vi "N4_X01.vi"(4 "error in":T15, 7 "Command":T16) -> (0 "error out":T15, 3 "Response":T13)   [LabVIEW 2018]
uses:
  MOKO_LabViewLibrary/MokoLowLevel/MokoLowLovelControl/MLLC_Command.ctl
  MOKO_LabViewLibrary/MokoLowLevel/MokoLowLovelControl/MLLC_Error.ctl
  MOKO_LabViewLibrary/MokoLowLevel/MokoLowLovelControl/MLLC_Mode.ctl
  MOKO_LabViewLibrary/MokoLowLevel/MokoLowLovelControl/MLLC_Response.ctl
  MOKO_LabViewLibrary/MokoLowLevel/MokoLowLovelControl/MLLC_DriverName.ctl
  MOKO_LabViewLibrary/MokoLowLevel/MokoLowLovelControl/MLLC_Request.ctl
  MOKO_LabViewLibrary/MokoLowLevel/MokoLowLovelControl/MLLC_ErrorCode.ctl
  MOKO_LabViewLibrary/MokoLowLevel/MokoLowLovelControl/MLLC_ResponseInit.ctl
  MOKO_LabViewLibrary/MokoLowLevel/MokoLowLovelControl/MLLC_ConnectCluster.ctl
  MOKO_LabViewLibrary/MokoLowLevel/MokoLowLovelControl/MLLC_InterfaceType.ctl
  MOKO_LabViewLibrary/MokoLowLevel/MokoLowLovelControl/MLLC_OpenedSession.ctl
  MOKO_LabViewLibrary/MokoLowLevel/MokoLowLovelControl/MLLC_InterfaceSettings.ctl
  MOKO_LabViewLibrary/MokoLowLevel/MokoLowLovelControl/MLLC_InterfaceKind.ctl
  MOKO_LabViewLibrary/MokoLowLevel/MokoLowLovelControl/MLLC_Boolean.ctl
  MOKO_LabViewLibrary/MokoLowLevel/MokoLowLovelControl/MLLC_Delay.ctl
panel:
  in  "Settings":T8={"Saved Data"=variant, "Permanent data"={"Connect"={"InterfaceType"=enum."VISA", "OpenedSession"="COM1", "InterfaceSettings"={"Interface"=enum."RS232", "EOS 4 read"=enum."LF (\\n)", "EOS 4 write"=enum."LF (\\n)", "TMO, ms"=10000, "Sett"=variant(cluster{"Baud Rate":u32, "Data Bits":u16, "Parity":u16, "Stop Bits":u16, "Flow Control":u16, "Eho":bool} {"Baud Rate"=75, "Data Bits"=0, "Parity"=0, "Stop Bits"=0, "Flow Control"=0, "Eho"=FALSE})}}, "RangeAuto"=TRUE, "SwitchOFF"=TRUE, "Range"=0.0}}
  in  "ResponseInit":T9="N4-101"
  in  "Error Code":T10=5470
  in  "Request":T11="IDN?"
  in  "Driver Name":T12="N4_101"
  in  "Mode":T14=enum."Check"
  # "Í4-X01"
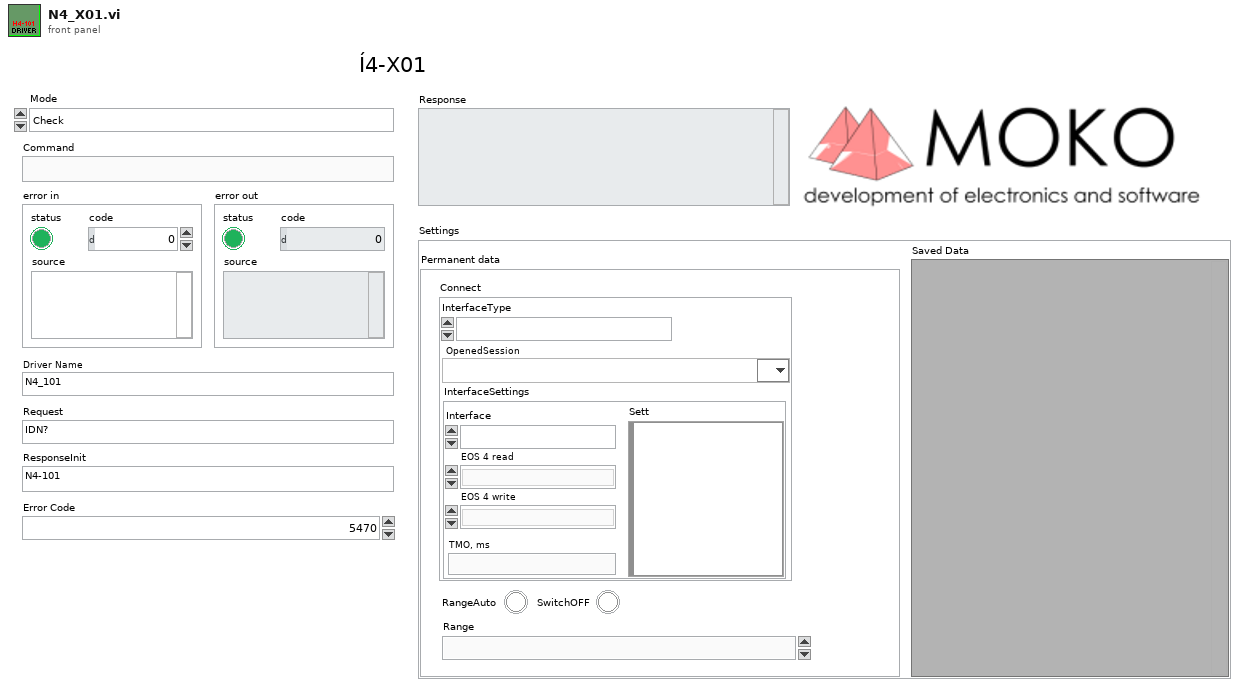
[diagram p1: front panel]
types:
  T1 = typedef "MLLC_ConnectCluster.ctl" = cluster{"InterfaceType":T2, "OpenedSession":T3, "InterfaceSettings":T4}
  T2 = typedef "MLLC_InterfaceType.ctl" = enum16{"VISA", "Prologix USB-GPIB"}
  T3 = typedef "MLLC_OpenedSession.ctl" = refnum<visa-resource-name>
  T4 = typedef "MLLC_InterfaceSettings.ctl" = cluster{"Interface":T5, "EOS 4 read":enum16{"Default (=EOS 4 write)", "CR (\\r)", "LF (\\n)", "None"}, "EOS 4 write":enum16{"CR+LF (\\r\\n)", "CR (\\r)", "LF (\\n)", "None"}, "TMO, ms":i32, "Sett":variant}
  T5 = typedef "MLLC_InterfaceKind.ctl" = enum16{"RS232", "GPIB", "USB", "Ethernet", "another"}
  T6 = typedef "MLLC_Boolean.ctl" = bool
  T7 = typedef "MLLC_Delay.ctl" = dbl
  T8 = cluster{"Saved Data":variant, "Permanent data":cluster{"Connect":T1, "RangeAuto":T6, "SwitchOFF":T6, "Range":T7}}
  T9 = typedef "MLLC_ResponseInit.ctl" = string
  T10 = typedef "MLLC_ErrorCode.ctl" = u32
  T11 = typedef "MLLC_Request.ctl" = string
  T12 = typedef "MLLC_DriverName.ctl" = string
  T13 = typedef "MLLC_Response.ctl" = string
  T14 = typedef "MLLC_Mode.ctl" = enum16{"get", "set", "close", "Init", "Check"}
  T15 = typedef "MLLC_Error.ctl" = errorcluster
  T16 = typedef "MLLC_Command.ctl" = string
  T17 = cluster{"Connect":T1, "RangeAuto":T6, "SwitchOFF":T6, "Range":T7}
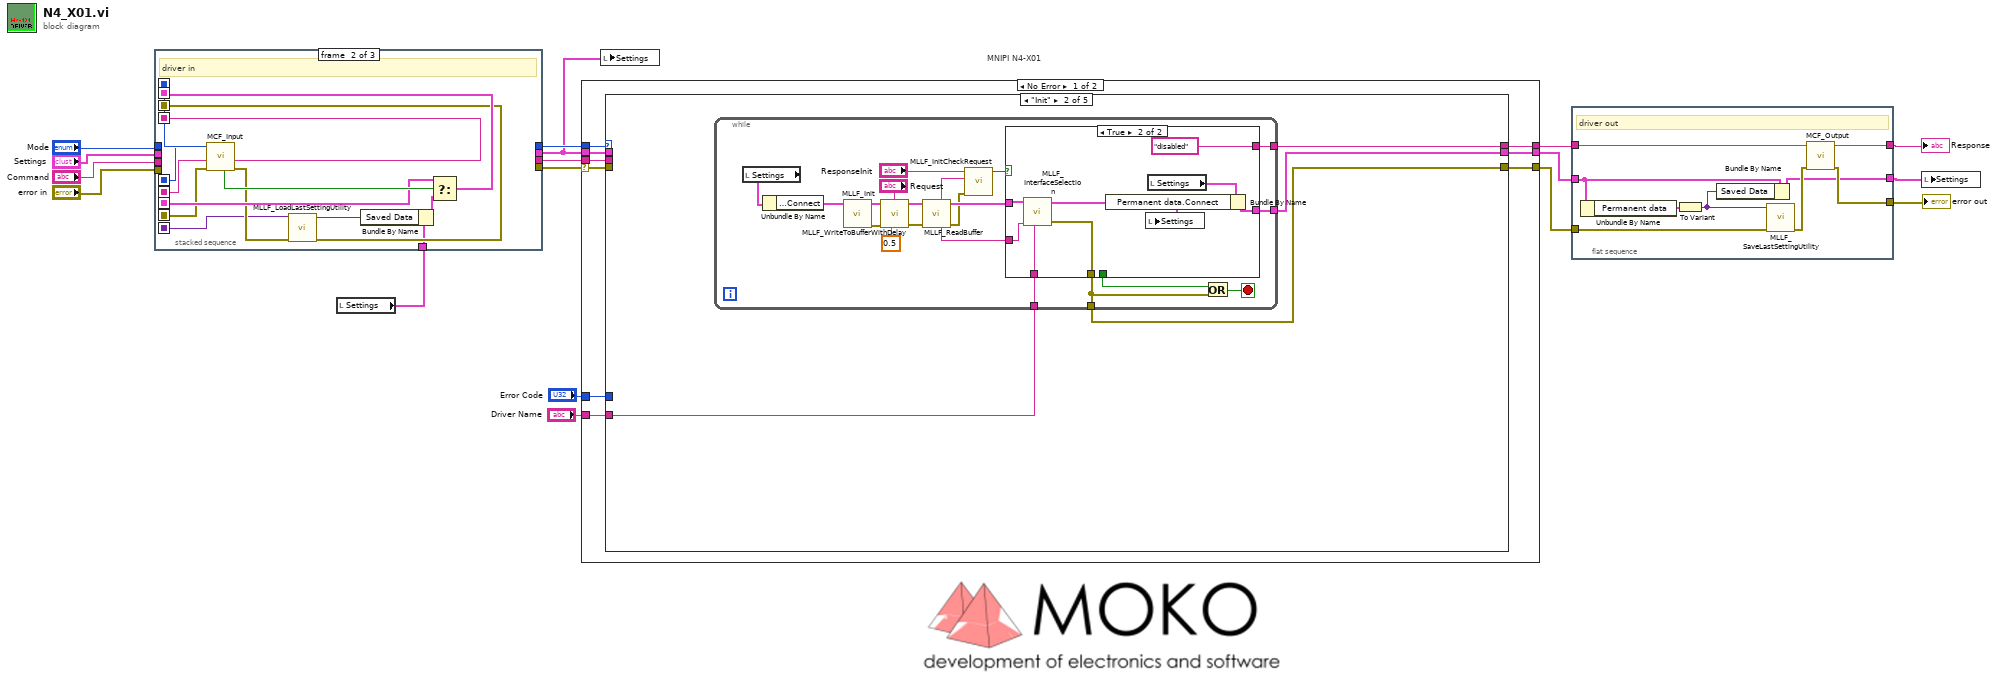
[diagram p0: block diagram]
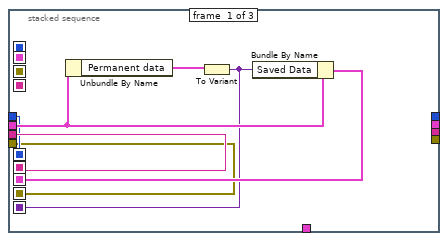
[diagram p2: hidden frame]
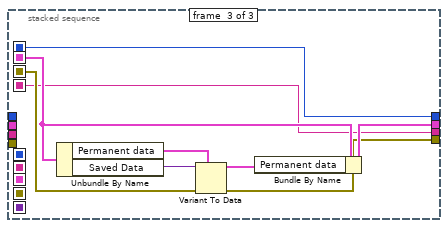
[diagram p3: hidden frame]
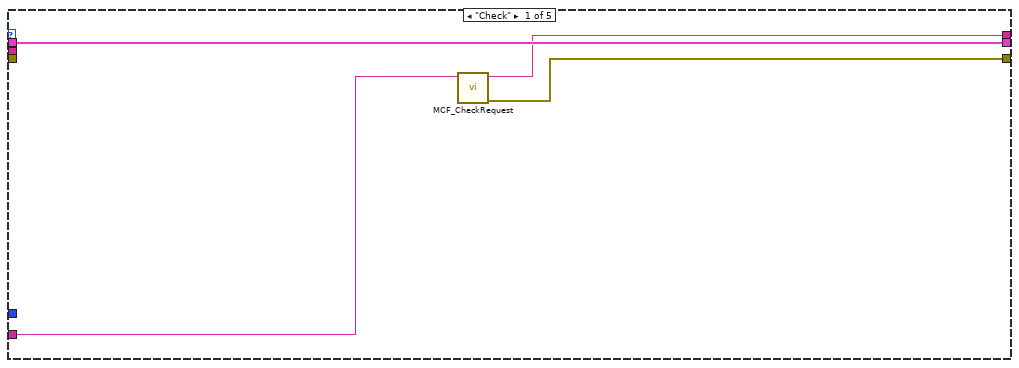
[diagram p4: hidden frame]
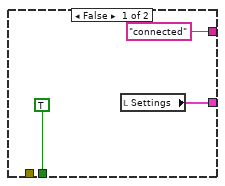
[diagram p5: hidden frame]
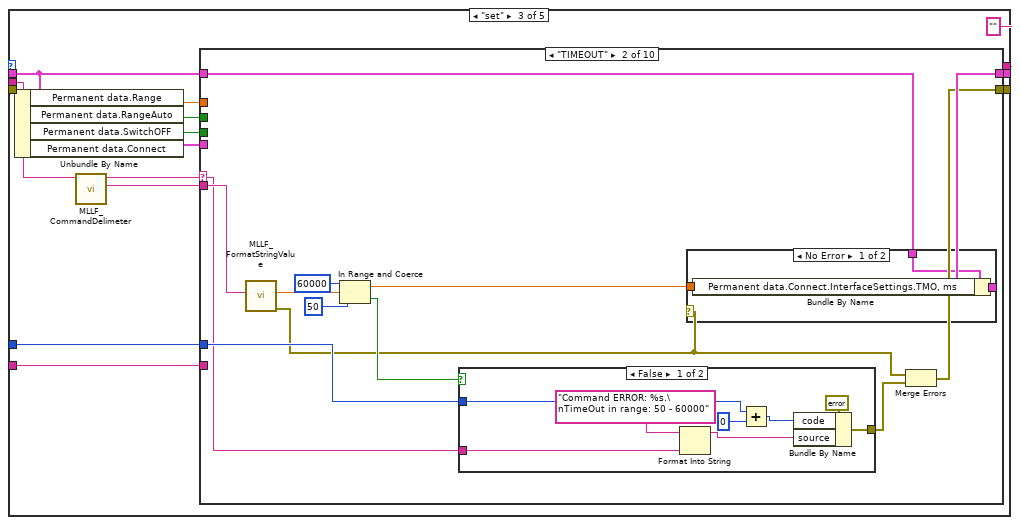
[diagram p6: hidden frame]
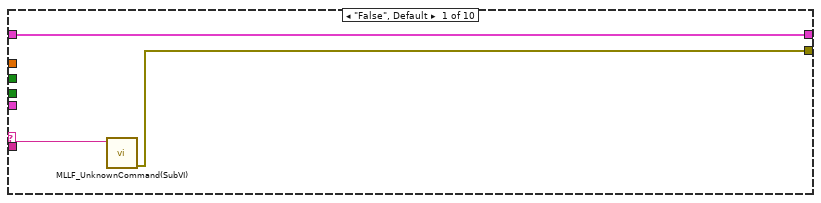
[diagram p7: hidden frame]
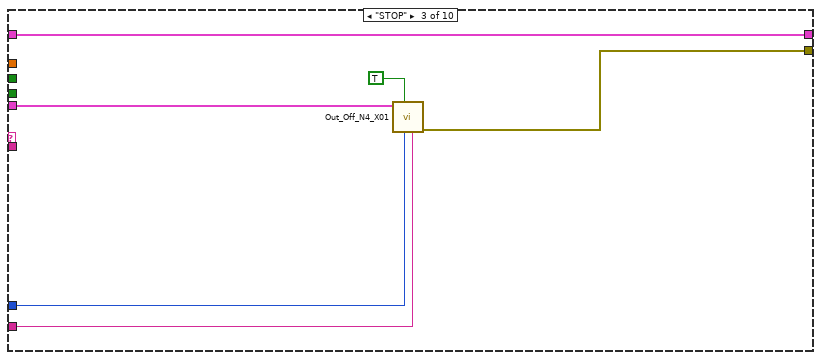
[diagram p10: hidden frame]
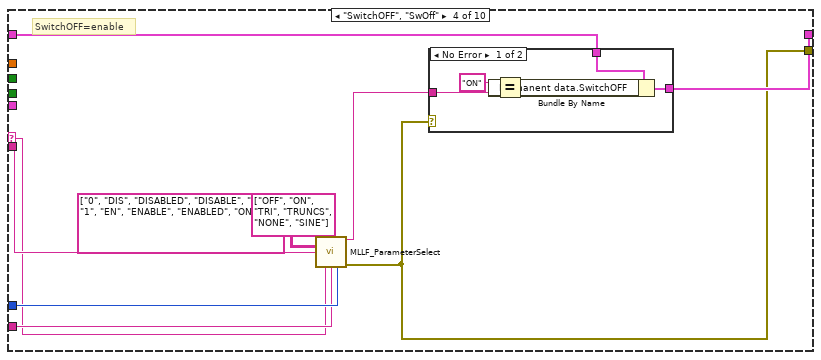
[diagram p11: hidden frame]
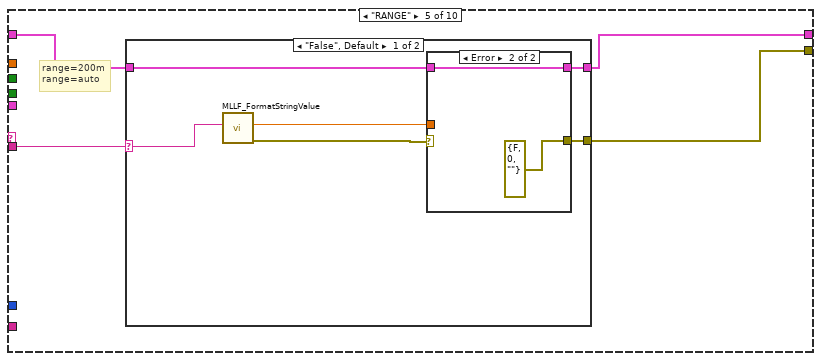
[diagram p13: hidden frame]
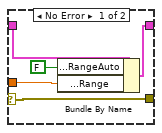
[diagram p14: hidden frame]
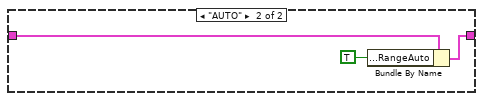
[diagram p15: hidden frame]
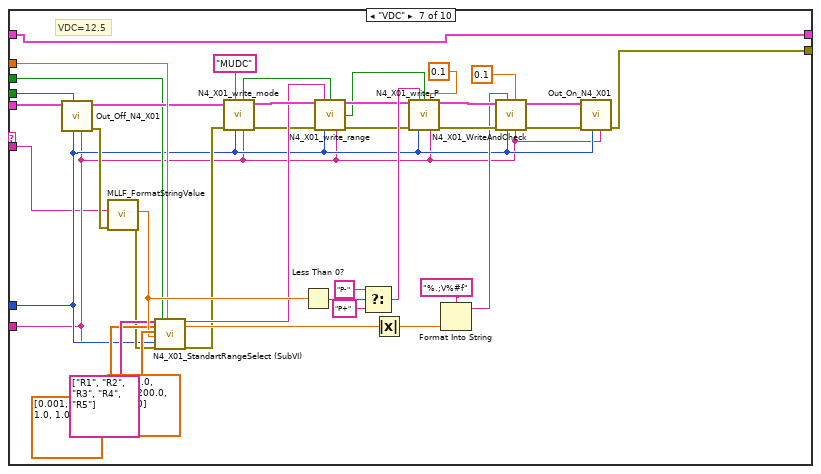
[diagram p17: hidden frame]
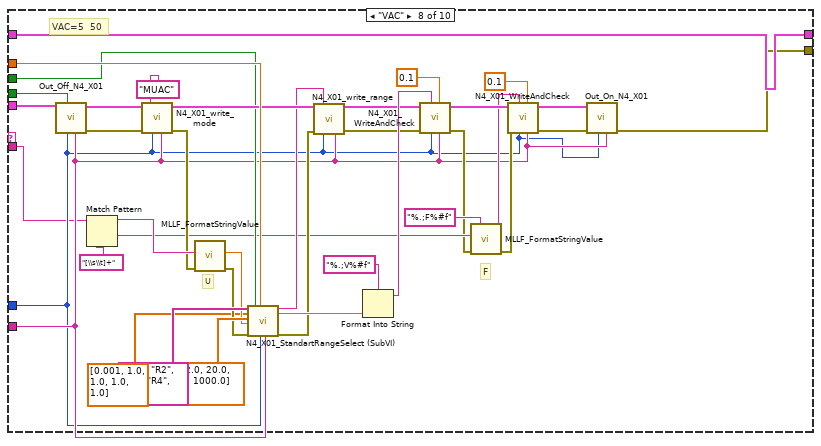
[diagram p18: hidden frame]
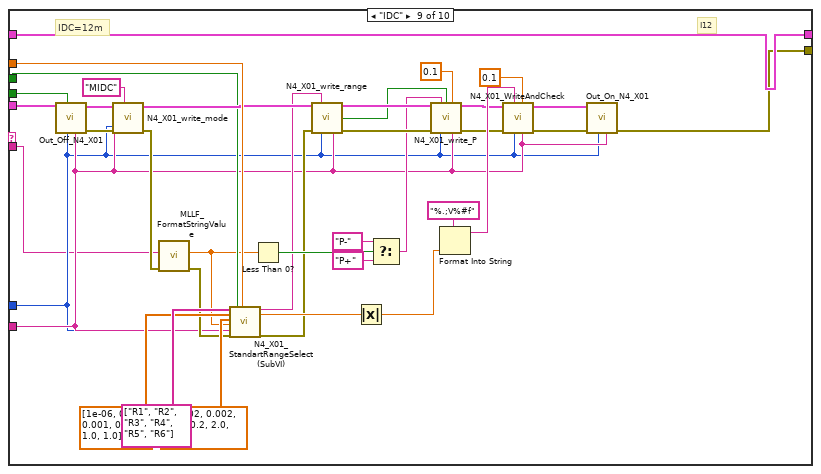
[diagram p19: hidden frame]
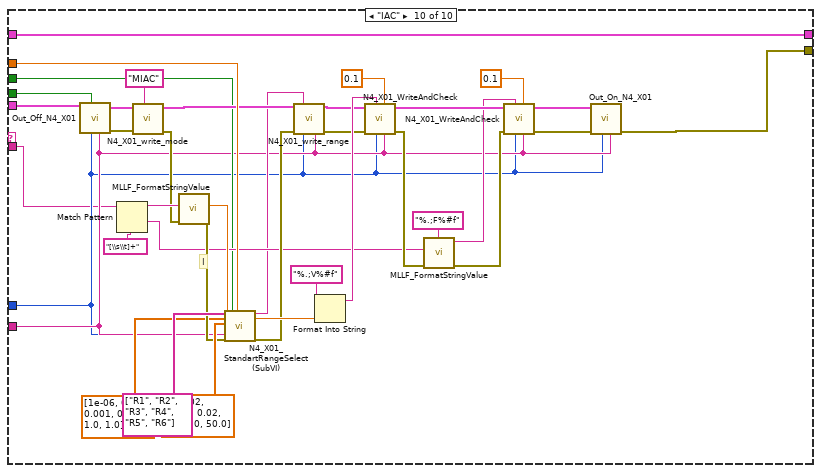
[diagram p20: hidden frame]
diagram:
  # "MNIPI N4-X01"
  n1 = local read "Settings"() -> (w7:T8)
  n2 = stacked-sequence {
    seq-local: [w20 _ _] -> [_ w36 _]
    seq-local: [w19 _ _] -> [_ w37 _]
    seq-local: [w22 _ _] -> [_ w32 _]
    seq-local: [w18 _ _] -> [_ w31 _]
    seq-local: [w21 _ _] -> [_ w27 _]
    seq-local: [_ w28 _] -> [_ _ w44]
    seq-local: [_ w38 _] -> [_ _ w41]
    seq-local: [_ w35 _] -> [_ _ w40]
    seq-local: [_ w34 _] -> [_ _ w45]
    tunnel: "Command" -> [w20 _ _]
    tunnel: "Mode" -> [w19 _ _]
    tunnel: "error in" -> [w18 _ _]
    tunnel: "Settings" -> [w23 _ _]
    tunnel: w7 -> [_ w26 _]
    tunnel: [_ _ w40] -> w9
    tunnel: [_ _ w43] -> w10
    tunnel: [_ _ w42] -> w8
    tunnel: [_ _ w41] -> w11
    frame #0 {
      n3 = Unbundle By Name(w23) -> ("Permanent data"=w24:T17)
      n4 = To Variant(anything=w24) -> (Variant=w21:variant)
      n5 = Bundle By Name(cluster=w23, "Saved Data"=w21) -> (w22:T8)
    }
    frame #1 {
      # "driver in"
      n6 = call "MCF_Input.vi"("Error In"=w31, "Command in"=w36, "Mode in"=w37) -> ("Error Out"=w30:errorcluster, "Command out"=w35:string, "Mode out"=w38:T14, "Boolean"=w33:bool)  [unwired: 5 in]
      n7 = call "MLLF_LoadLastSettingUtility.vi"("Error In"=w30, "Save data in"=w27) -> ("Error Out"=w28:errorcluster, "Save data out"=w25:variant)  [unwired: 8 in]
      n8 = Bundle By Name(cluster=w26, "Saved Data"=w25) -> (w29:T8)
      n9 = Select(t=w32, s=w33, f=w29) -> (s? t:f=w34:T8)
    }
    frame #2 {
      n10 = Unbundle By Name(w45) -> ("Permanent data"=w46:T17, "Saved Data"=w39:variant)
      n11 = Variant To Data(error in=w44, type=w46, Variant=w39) -> (data=w47:T17, error out=w42:errorcluster)
      n12 = Bundle By Name(cluster=w45, "Permanent data"=w47) -> (w43:T8)
    }
  }
  n13 = case shown="No Error" w8 {
    selector: w8 -> [w52 w371]
    tunnel: [w54 w371] -> w4
    tunnel: w11 -> [w56 _]
    tunnel: [w55 "" ("String")] -> w6
    tunnel: w9 -> [w53 _]
    tunnel: w10 -> [w49 w370]
    tunnel: "Error Code" -> [w51 _]
    tunnel: "Driver Name" -> [w50 _]
    tunnel: [w48 w370] -> w5
    frame No Error {
      n14 = case shown="\"Init\"" w56 {
        tunnel: [w58 w64 "" ("String") w333 "" ("String")] -> w55
        tunnel: [w59 w62 w97 w332 w367] -> w54
        tunnel: w53 -> [_ _ w107 w343 _]
        tunnel: w52 -> [_ _ _ _ _]
        tunnel: w51 -> [_ _ w106 w340 _]
        tunnel: w50 -> [w57 w61 w103 w339 _]
        tunnel: w49 -> [w60 _ w105 w342 w366]
        tunnel: [w60 w63 w104 w341 w366] -> w48
        frame "Check" {
          n15 = call "MCF_CheckRequest.vi"("Driver Name"=w57) -> ("Error Out"=w59:errorcluster, "Output String"=w58:string)  [unwired: 9 in]
        }
        frame "Init" {
          n16 = while {
            tunnel: [w76] -> w62
            tunnel: [w68] -> w63
            tunnel: [w67] -> w64
            tunnel: w61 -> [w66]
            stop <- w74 stop-if-true
            n17 = local read "Settings"() -> (w83:T8)
            n18 = Unbundle By Name(w83) -> ("Permanent data.Connect"=w77:T1)
            n19 = call "MLLF_Init.vi"("DriverConnect in"=w77) -> ("Error Out"=w79:errorcluster, "DriverConnect out"=w78:T1)  [unwired: 7 in]
            n20 = call "MLLF_WriteToBufferWithDelay.vi"("Delay Time ( 0,05 s)"=0.5 ("Delay Time (s)"), "Command"="Request", "Error In"=w79, "DriverConnect in"=w78) -> ("Error Out"=w72:errorcluster, "DriverConnect out"=w81:T1)  [unwired: 6 in]
            n21 = call "MLLF_ReadBuffer.vi"("Error In"=w72, "DriverConnect in"=w81) -> ("Error Out"=w70:errorcluster, "DriverConnect out"=w80:T1, "String"=w65:string)  [unwired: 6 in]
            n22 = call "MLLF_InitCheckRequest.vi"("error in (no error)"=w70, "Answer"=w65, "Response Init"="ResponseInit") -> ("Design"=w69:bool)  [unwired: 5 in, 3 out]
            n23 = case shown="True" w69 {
              tunnel: w80 -> [_ w93]
              tunnel: [_ w94] -> w76
              tunnel: [TRUE _] -> w75
              tunnel: [w84 w90] -> w68
              tunnel: ["connected" "disabled"] -> w67
              tunnel: w66 -> [_ w88]
              tunnel: w65 -> [_ w87]
              frame False {
                n24 = local read "Settings"() -> (w84:T8)
              }
              frame True {
                n25 = call "MLLF_InterfaceSelection.vi"("Driver Name"=w88, "Answer:"=w87, "DriverConnect in"=w93) -> ("error out"=w94:T15, "DriverConnect out"=w92:T1)  [unwired: 4 in, 3 out]
                n26 = local read "Settings"() -> (w91:T8)
                n27 = Bundle By Name(cluster=w91, "Permanent data.Connect"=w92) -> (w90:T8)
                n28 = local write "Settings"(w90) -> ()
              }
            }
            n29 = Or(x=w75, y=w76) -> (x .or. y?=w74:bool)
          }
        }
        frame "set" {
          n30 = Unbundle By Name(w105) -> ("Permanent data.Range"=w98:T7, "Permanent data.RangeAuto"=w99:T6, "Permanent data.SwitchOFF"=w100:T6, "Permanent data.Connect"=w101:T1)
          n31 = call "MLLF_CommandDelimeter.vi"("command with param"=w107) -> ("param 1"=w95:string, "command"=w96:string)  [unwired: 6 in, 3 out]
          n32 = case shown="\"TIMEOUT\"" w96 {
            selector: w96 -> [w109 w111 _ w142 _ _ _ _ _ _]
            tunnel: w95 -> [_ w114 _ w143 w161 _ w179 w219 w256 w295]
            tunnel: [w108 w117 w140 w146 w160 _ w180 w218 w257 w294] -> w97
            tunnel: w106 -> [_ w118 w138 w145 _ _ w183 w220 w259 w296]
            tunnel: w105 -> [w110 w122 w141 w148 w159 w178 w217 w254 w292 w330]
            tunnel: [w110 w123 w141 w147 w158 w178 w217 w254 w292 w330] -> w104
            tunnel: w101 -> [_ _ w137 _ _ _ w201 w255 w293 w331]
            tunnel: w103 -> [_ _ w139 w144 _ _ w182 w221 w260 w297]
            tunnel: w100 -> [_ _ _ _ _ _ w200 w246 w287 w321]
            tunnel: w99 -> [_ _ _ _ _ _ w194 w232 w267 w302]
            tunnel: w98 -> [_ _ _ _ _ _ w202 w238 w279 w313]
            frame "False", Default {
              n33 = call "MLLF_UnknownCommand(SubVI).vi"("Unknown command"=w109) -> ("error out"=w108:errorcluster)  [unwired: 10 in]
            }
            frame "TIMEOUT" {
              n34 = call "MLLF_FormatStringValue.vi"("String Value"=w114) -> ("error out"=w112:T15, "number"=w113:dbl)  [unwired: 8 in, 1 out]
              n35 = In Range and Coerce(upper limit=60000, x=w113, lower limit=50) -> (coerced(x)=w119:dbl, In Range?=w115:bool)
              n36 = case shown="False" w115 {
                tunnel: [w130 _] -> w116
                tunnel: w118 -> [w129 _]
                tunnel: w111 -> [w128 _]
                frame False {
                  n37 = Format Into String(format string="Command ERROR: %s.\nTimeOut in range: 50 - 60000", w128) -> (resulting string=w132:string)  [unwired: 2 in, 1 out]
                  n38 = Add(x=w129, y=0) -> (x+y=w133:T10)
                  n39 = Bundle By Name(cluster=errorcluster {"status"=TRUE, "code"=0, "source"=""} ("error out"), "code"=w133, "source"=w132) -> (w130:errorcluster)
                }
                frame True {
                }
              }
              n40 = case shown="No Error" w112 {
                tunnel: [w126 w127] -> w123
                tunnel: w122 -> [w125 w127]
                tunnel: w119 -> [w124 _]
                frame No Error {
                  n41 = Bundle By Name(cluster=w125, "Permanent data.Connect.InterfaceSettings.TMO, ms"=w124) -> (w126:T8)
                }
                frame Error {
                }
              }
              n42 = Merge Errors(w112, w116) -> (w117:errorcluster)
            }
            frame "STOP" {
              n43 = call "Out_Off_N4_X01.vi"("Driver Name"=w139, "Error Code"=w138, "SwitchOFF"=TRUE, "DriverConnect in"=w137) -> ("error out"=w140:T15)  [unwired: 6 in, 1 out]
            }
            frame "SwitchOFF", "SwOff" {
              # "SwitchOFF=enable"
              n44 = call "MLLF_ParameterSelect.vi"("Command to equipment"=string[] ["OFF", "ON", "TRI", "TRUNCS", "NONE", "SINE"] ("Parameters"), "Names"=string[][] [["0", "DIS", "DISABLED", "DISABLE", "OFF"], ["1", "EN", "ENABLE", "ENABLED", "ON"]], "Input"=w143, "Command"=w142, "Driver Name"=w144, "Error Code"=w145) -> ("Choice"=w151:string, "Error Out"=w146:errorcluster)  [unwired: 8 in]
              n45 = case shown="No Error" w146 {
                tunnel: w151 -> [w156 _]
                tunnel: w148 -> [w154 w157]
                tunnel: [w153 w157] -> w147
                frame No Error {
                  n46 = Equal?(x="ON", y=w156) -> (x = y?=w152:bool)
                  n47 = Bundle By Name(cluster=w154, "Permanent data.SwitchOFF"=w152) -> (w153:T8)
                }
                frame Error {
                }
              }
            }
            frame "RANGE" {
              # "range=200m\nrange=auto"
              n48 = case shown="\"False\", Default" w161 {
                selector: w161 -> [w167 _]
                tunnel: [w162 _] -> w160
                tunnel: [w165 w177] -> w158
                tunnel: w159 -> [w166 w176]
                frame "False", Default {
                  n49 = call "MLLF_FormatStringValue.vi"("String Value"=w167) -> ("error out"=w163:T15, "number"=w164:dbl)  [unwired: 8 in, 1 out]
                  n50 = case shown="Error" w163 {
                    selector: w163 -> [w168 _]
                    tunnel: w166 -> [w171 w174]
                    tunnel: [w170 w174] -> w165
                    tunnel: w164 -> [w169 _]
                    tunnel: [w168 errorcluster {"status"=FALSE, "code"=0, "source"=""} ("error IO")] -> w162
                    frame No Error {
                      n51 = Bundle By Name(cluster=w171, "Permanent data.RangeAuto"=FALSE ("RangeAuto"), "Permanent data.Range"=w169) -> (w170:T8)
                    }
                    frame Error {
                    }
                  }
                }
                frame "AUTO" {
                  n52 = Bundle By Name(cluster=w176, "Permanent data.RangeAuto"=TRUE ("RangeAuto")) -> (w177:T8)
                }
              }
            }
            frame "<----MAIN FUNCTIONS---->" {
            }
            frame "VDC" {
              # "VDC=12.5"
              n53 = call "Out_Off_N4_X01.vi"("Driver Name"=w182, "Error Code"=w183, "SwitchOFF"=w200, "DriverConnect in"=w201) -> ("error out"=w190:T15, "DriverConnect out"=w196:T1)  [unwired: 6 in]
              n54 = call "MLLF_FormatStringValue.vi"("error in"=w190, "String Value"=w179) -> ("error out"=w192:T15, "number"=w215:dbl)  [unwired: 7 in, 1 out]
              n55 = call "N4_X01_StandartRangeSelect (SubVI).vi"("Range Command"=string[] ["R1", "R2", "R3", "R4", "R5"] ("RangeCommand"), "Scale Array"=dbl[] [0.001, 1.0, 1.0, 1.0, 1.0] ("ScaleArray"), "Range Digit"=dbl[] [0.2, 2.0, 20.0, 200.0, 1000.0] ("RangeDigit"), "Control Point"=w215, "Error In"=w192, "RangeAuto"=w194, "Range"=w202, "Error Code"=w183, "Driver Name"=w182) -> ("Range Out"=w195:string, "Scaled value"=w213:dbl, "Error Out"=w189:errorcluster)  [unwired: 8 in]
              n56 = call "N4_X01_write_mode.vi"("Driver Name"=w182, "Error Code"=w183, "Command"="MUDC" ("String"), "error in"=w189, "DriverConnect in"=w196) -> ("error out"=w188:T15, "DriverConnect out"=w199:T1, "ModeWasChacged"=w187:T6)  [unwired: 4 in]
              n57 = Less Than 0?(x=w215) -> (x < 0?=w212:bool)
              n58 = call "N4_X01_write_range.vi"("DriverConnect in"=w199, "Command range"=w195, "ModeIsChanged?"=w187, "error in"=w188, "Error Code"=w183, "Driver Name"=w182) -> ("DriverConnect out"=w198:T1, "RangeWasChanged"=w191:T6, "error out"=w197:T15)  [unwired: 7 in]
              n59 = Select(t="P-" ("String"), s=w212, f="P+" ("String")) -> (s? t:f=w209:string)
              n60 = Absolute Value(x=w213) -> (abs(x)=w206:dbl)
              n61 = call "N4_X01_write_P.vi"("DriverConnect in"=w198, "P"=w209, "RangeIsChanged?"=w191, "Command Time (s)"=0.1, "error in"=w197, "Error Code"=w183, "Driver Name"=w182) -> ("DriverConnect out"=w207:T1, "error out"=w208:T15)  [unwired: 7 in]
              n62 = Format Into String(format string="%.;V%#f", w206) -> (resulting string=w204:string)  [unwired: 2 in, 1 out]
              n63 = call "N4_X01_WriteAndCheck.vi"("Driver Name"=w182, "Command Time (s)"=0.1, "Error Code"=w183, "Command"=w204, "error in"=w208, "DriverConnect in"=w207) -> ("error out"=w184:T15, "DriverConnect out"=w185:T1)  [unwired: 4 in]
              n64 = call "Out_On_N4_X01.vi"("Driver Name"=w182, "Error Code"=w183, "error in"=w184, "DriverConnect in"=w185) -> ("error out"=w180:T15)  [unwired: 6 in, 1 out]
            }
            frame "VAC" {
              # "VAC=5  50"
              # "F"
              # "U"
              n65 = call "Out_Off_N4_X01.vi"("Driver Name"=w221, "Error Code"=w220, "SwitchOFF"=w246, "DriverConnect in"=w255) -> ("error out"=w231:T15, "DriverConnect out"=w237:T1)  [unwired: 6 in]
              n66 = Match Pattern(string=w219, regular expression="[\\s\\t]+") -> (before substring=w239:string, after substring=w228:string)  [unwired: 1 in, 2 out]
              n67 = call "N4_X01_write_mode.vi"("Driver Name"=w221, "Error Code"=w220, "Command"="MUAC" ("String"), "error in"=w231, "DriverConnect in"=w237) -> ("error out"=w230:T15, "DriverConnect out"=w236:T1)  [unwired: 4 in, 1 out]
              n68 = call "MLLF_FormatStringValue.vi"("error in"=w230, "String Value"=w239) -> ("error out"=w248:T15, "number"=w249:dbl)  [unwired: 7 in, 1 out]
              n69 = call "N4_X01_StandartRangeSelect (SubVI).vi"("Range Command"=string[] ["R1", "R2", "R3", "R4", "R5"] ("RangeCommand"), "Scale Array"=dbl[] [0.001, 1.0, 1.0, 1.0, 1.0] ("ScaleArray"), "Range Digit"=dbl[] [0.2, 2.0, 20.0, 200.0, 1000.0] ("RangeDigit"), "Control Point"=w249, "Error In"=w248, "RangeAuto"=w232, "Range"=w238, "Error Code"=w220, "Driver Name"=w221) -> ("Range Out"=w235:string, "Scaled value"=w243:dbl, "Error Out"=w229:errorcluster)  [unwired: 8 in]
              n70 = call "N4_X01_write_range.vi"("DriverConnect in"=w236, "Command range"=w235, "error in"=w229, "Error Code"=w220, "Driver Name"=w221) -> ("DriverConnect out"=w234:T1, "error out"=w233:T15)  [unwired: 8 in, 1 out]
              n71 = Format Into String(format string="%.;V%#f", w243) -> (resulting string=w240:string)  [unwired: 2 in, 1 out]
              n72 = call "N4_X01_WriteAndCheck.vi"("Driver Name"=w221, "Command Time (s)"=0.1, "Error Code"=w220, "Command"=w240, "error in"=w233, "DriverConnect in"=w234) -> ("error out"=w227:T15, "DriverConnect out"=w245:T1)  [unwired: 4 in]
              n73 = call "MLLF_FormatStringValue.vi"("error in"=w227, "String Value"=w228, "Format"="%.;F%#f" ("format string")) -> ("error out"=w244:T15, "String Value Formated"=w241:T16)  [unwired: 6 in, 1 out]
              n74 = call "N4_X01_WriteAndCheck.vi"("Driver Name"=w221, "Command Time (s)"=0.1, "Error Code"=w220, "Command"=w241, "error in"=w244, "DriverConnect in"=w245) -> ("error out"=w222:T15, "DriverConnect out"=w223:T1)  [unwired: 4 in]
              n75 = call "Out_On_N4_X01.vi"("Driver Name"=w221, "Error Code"=w220, "error in"=w222, "DriverConnect in"=w223) -> ("error out"=w218:T15)  [unwired: 6 in, 1 out]
            }
            frame "IDC" {
              # "IDC=12m"
              # "I12"
              n76 = call "Out_Off_N4_X01.vi"("Driver Name"=w260, "Error Code"=w259, "SwitchOFF"=w287, "DriverConnect in"=w293) -> ("error out"=w271:T15, "DriverConnect out"=w273:T1)  [unwired: 6 in]
              n77 = call "N4_X01_write_mode.vi"("Driver Name"=w260, "Error Code"=w259, "Command"="MIDC" ("String"), "error in"=w271, "DriverConnect in"=w273) -> ("error out"=w270:T15, "DriverConnect out"=w276:T1)  [unwired: 4 in, 1 out]
              n78 = call "MLLF_FormatStringValue.vi"("error in"=w270, "String Value"=w256) -> ("error out"=w286:T15, "number"=w264:dbl)  [unwired: 7 in, 1 out]
              n79 = call "N4_X01_StandartRangeSelect (SubVI).vi"("Range Command"=string[] ["R1", "R2", "R3", "R4", "R5", "R6"] ("RangeCommand"), "Scale Array"=dbl[] [1e-06, 0.001, 0.001, 0.001, 1.0, 1.0] ("ScaleArray"), "Range Digit"=dbl[] [0.0002, 0.002, 0.02, 0.2, 2.0, 50.0] ("RangeDigit"), "Control Point"=w264, "Error In"=w286, "RangeAuto"=w267, "Range"=w279, "Error Code"=w259, "Driver Name"=w260) -> ("Range Out"=w272:string, "Scaled value"=w288:dbl, "Error Out"=w269:errorcluster)  [unwired: 8 in]
              n80 = Less Than 0?(x=w264) -> (x < 0?=w283:bool)
              n81 = call "N4_X01_write_range.vi"("DriverConnect in"=w276, "Command range"=w272, "error in"=w269, "Error Code"=w259, "Driver Name"=w260) -> ("DriverConnect out"=w277:T1, "RangeWasChanged"=w265:T6, "error out"=w278:T15)  [unwired: 8 in]
              n82 = Absolute Value(x=w288) -> (abs(x)=w280:dbl)
              n83 = Select(t="P-" ("String"), s=w283, f="P+" ("String")) -> (s? t:f=w268:string)
              n84 = call "N4_X01_write_P.vi"("DriverConnect in"=w277, "P"=w268, "RangeIsChanged?"=w265, "Command Time (s)"=0.1, "error in"=w278, "Error Code"=w259, "Driver Name"=w260) -> ("DriverConnect out"=w275:T1, "error out"=w274:T15)  [unwired: 7 in]
              n85 = Format Into String(format string="%.;V%#f", w280) -> (resulting string=w282:string)  [unwired: 2 in, 1 out]
              n86 = call "N4_X01_WriteAndCheck.vi"("Driver Name"=w260, "Command Time (s)"=0.1, "Error Code"=w259, "Command"=w282, "error in"=w274, "DriverConnect in"=w275) -> ("error out"=w261:T15, "DriverConnect out"=w262:T1)  [unwired: 4 in]
              n87 = call "Out_On_N4_X01.vi"("Driver Name"=w260, "Error Code"=w259, "error in"=w261, "DriverConnect in"=w262) -> ("error out"=w257:T15)  [unwired: 6 in, 1 out]
            }
            frame "IAC" {
              # "I"
              n88 = call "Out_Off_N4_X01.vi"("Driver Name"=w297, "Error Code"=w296, "SwitchOFF"=w321, "DriverConnect in"=w331) -> ("error out"=w307:T15, "DriverConnect out"=w309:T1)  [unwired: 6 in]
              n89 = Match Pattern(string=w295, regular expression="[\\s\\t]+") -> (before substring=w328:string, after substring=w304:string)  [unwired: 1 in, 2 out]
              n90 = call "N4_X01_write_mode.vi"("Command"="MIAC" ("String"), "error in"=w307, "DriverConnect in"=w309) -> ("error out"=w306:T15, "DriverConnect out"=w312:T1)  [unwired: 6 in, 1 out]
              n91 = call "MLLF_FormatStringValue.vi"("error in"=w306, "String Value"=w328) -> ("error out"=w324:T15, "number"=w323:dbl)  [unwired: 7 in, 1 out]
              n92 = call "N4_X01_StandartRangeSelect (SubVI).vi"("Range Command"=string[] ["R1", "R2", "R3", "R4", "R5", "R6"] ("RangeCommand"), "Scale Array"=dbl[] [1e-06, 0.001, 0.001, 0.001, 1.0, 1.0] ("ScaleArray"), "Range Digit"=dbl[] [0.0002, 0.002, 0.02, 0.2, 2.0, 50.0] ("RangeDigit"), "Control Point"=w323, "Error In"=w324, "RangeAuto"=w302, "Range"=w313, "Error Code"=w296, "Driver Name"=w297) -> ("Range Out"=w303:string, "Scaled value"=w316:dbl, "Error Out"=w305:errorcluster)  [unwired: 8 in]
              n93 = call "N4_X01_write_range.vi"("DriverConnect in"=w312, "Command range"=w303, "error in"=w305, "Error Code"=w296, "Driver Name"=w297) -> ("DriverConnect out"=w311:T1, "error out"=w310:T15)  [unwired: 8 in, 1 out]
              n94 = Format Into String(format string="%.;V%#f", w316) -> (resulting string=w320:string)  [unwired: 2 in, 1 out]
              n95 = call "N4_X01_WriteAndCheck.vi"("Driver Name"=w297, "Command Time (s)"=0.1, "Error Code"=w296, "Command"=w320, "error in"=w310, "DriverConnect in"=w311) -> ("error out"=w315:T15, "DriverConnect out"=w319:T1)  [unwired: 4 in]
              n96 = call "MLLF_FormatStringValue.vi"("error in"=w315, "String Value"=w304, "Format"="%.;F%#f" ("format string")) -> ("error out"=w314:T15, "String Value Formated"=w318:T16)  [unwired: 6 in, 1 out]
              n97 = call "N4_X01_WriteAndCheck.vi"("Driver Name"=w297, "Command Time (s)"=0.1, "Error Code"=w296, "Command"=w318, "error in"=w314, "DriverConnect in"=w319) -> ("error out"=w298:T15, "DriverConnect out"=w299:T1)  [unwired: 4 in]
              n98 = call "Out_On_N4_X01.vi"("Driver Name"=w297, "Error Code"=w296, "error in"=w298, "DriverConnect in"=w299) -> ("error out"=w294:T15)  [unwired: 6 in, 1 out]
            }
          }
        }
        frame "get" {
          n99 = Unbundle By Name(w342) -> ("Permanent data.Connect"=w336:T1)
          n100 = call "MLLF_CommandDelimeter.vi"("command with param"=w343) -> ("param 1"=w334:string, "command"=w335:string)  [unwired: 6 in, 3 out]
          n101 = case shown="\"AMPL\", \"AMPLITUDE\"" w335 {
            selector: w335 -> [w345 _ _]
            tunnel: w334 -> [_ _ _]
            tunnel: [w344 _ w353] -> w338
            tunnel: w340 -> [_ _ _]
            tunnel: [w348 w351 w364] -> w341
            tunnel: w342 -> [w348 w351 w364]
            tunnel: [w346 w349 w363] -> w337
            tunnel: w336 -> [_ _ w356]
            tunnel: w339 -> [_ _ _]
            frame "False", Default {
              n102 = call "MLLF_UnknownCommand(SubVI).vi"("Unknown command"=w345) -> ("error out"=w344:errorcluster)  [unwired: 10 in]
              n103 = Build Array(0 ("TimeOut")) -> (w346:i32[])
            }
            frame "TIMEOUT" {
              n104 = Unbundle By Name(w351) -> ("Permanent data.Connect.InterfaceSettings.TMO, ms"=w350:i32)
              n105 = Build Array(w350) -> (w349:i32[])
            }
            frame "AMPL", "AMPLITUDE" {
              n106 = call "MLLF_WriteToBuffer.vi"("String"="V?" ("Error Query"), "DriverConnect in"=w356) -> ("error out"=w361:T15, "DriverConnect out"=w357:T1)  [unwired: 6 in]
              n107 = call "500ms12"("error in (no error)"=w361, "Delay Time (s)"=0.5) -> ("error out"=w362:errorcluster)  [unwired: 9 in]
              n108 = call "MLLF_ReadBuffer.vi"("Error In"=w362, "DriverConnect in"=w357) -> ("Error Out"=w354:errorcluster, "String"=w359:string)  [unwired: 6 in, 1 out]
              n109 = call "MLLF_FormatStringValue.vi"("error in"=w354, "String Value"=w359, "Format"="%#e" ("format string")) -> ("error out"=w353:T15, "number"=w355:dbl)  [unwired: 6 in, 1 out]
              n110 = Build Array(w355) -> (w363:dbl[])
            }
          }
          n111 = call "MLLF_FormatOutputValueWithUnits.vi"("error in"=w338, "ValuesIn"=w337) -> ("error out"=w332:T15, "Result string"=w333:T16)  [unwired: 8 in]
        }
        frame "close" {
          n112 = Unbundle By Name(w366) -> ("Permanent data.Connect.OpenedSession"=w368:T3)
          n113 = VISA Close(VISA resource name=w368) -> (error out=w367:errorcluster)  [unwired: 1 in]
        }
      }
    }
    frame Error {
    }
  }
  n114 = local write "Settings"(w10) -> ()
  n115 = flat-sequence {
    tunnel: [w380] -> w1
    tunnel: [w379] -> w3
    tunnel: w6 -> [w378]
    tunnel: w4 -> [w377]
    tunnel: w5 -> [w373]
    tunnel: [w375] -> w2
    frame #0 {
      # "driver out"
      n116 = Unbundle By Name(w373) -> ("Permanent data"=w372:T17)
      n117 = To Variant(anything=w372) -> (Variant=w374:variant)
      n118 = Bundle By Name(cluster=w373, "Saved Data"=w374) -> (w375:T8)
      n119 = call "MLLF_SaveLastSettingUtility.vi"("error in"=w377, "Saved Data"=w374) -> ("error out"=w376:T15)  [unwired: 8 in, 1 out]
      n120 = call "MCF_Output.vi"("Error In"=w376, "Input"=w378) -> ("Error Out"=w379:errorcluster, "Output"=w380:string)  [unwired: 8 in]
    }
  }
  n121 = local write "Settings"(w2) -> ()
  "error out" <- w3
  "Response" <- w1
